vi "Log Folder.vi"(8 "error in (no error)":errorcluster, 11 "Node Config in":refnum<class "Node Config.lvclass">) -> (0 "error out":errorcluster, 2 "Log Folder":path, 3 "Node Config out":refnum<class "Node Config.lvclass">)   [LabVIEW 2020, in "VolatusConfig.lvlib" / "Node Config.lvclass"]
uses:
  Node Config.lvclass
  Node Config.lvclass/Node Config.ctl
  VolatusConfigElement/VolatusConfigElement.lvclass
  lv-cdm/CDM-Config/Config Element/Config Element.lvclass
  C:/dev/lv20CE/relink/lv-volatus/VolatusConfig/VolatusConfigElement/VolatusConfigElement.lvclass
  C:/dev/lv20CE/relink/lv-volatus/VolatusConfig/Node/Node Config.lvclass
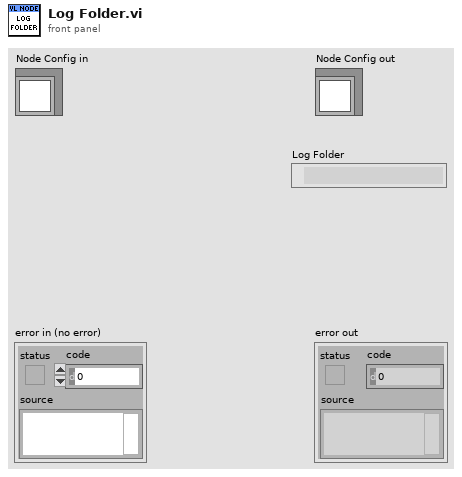
[diagram p1: front panel]
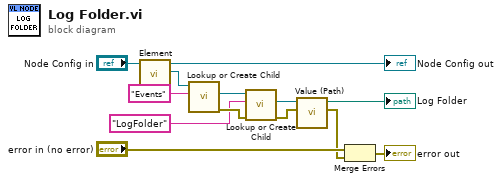
[diagram p0: block diagram]
diagram:
  n1 = call "Element.vi"("VolatusConfigElement in"="Node Config in") -> ("Element"=w12:refnum<class "Config Element.lvclass">, "VolatusConfigElement out"=→"Node Config out":refnum<class "Node Config.lvclass">)  [unwired: 9 in]
  n2 = call "Lookup or Create Child.vi"("Name"="Events", "Config Element in"=w12) -> ("error out"=w9:errorcluster, "Child"=w10:refnum<class "Config Element.lvclass">)  [unwired: 6 in, 2 out]
  n3 = call "Lookup or Create Child.vi"("error in (no error)"=w9, "Name"="LogFolder", "Config Element in"=w10) -> ("error out"=w7:errorcluster, "Child"=w6:refnum<class "Config Element.lvclass">)  [unwired: 5 in, 2 out]
  n4 = call "Value (Path).vi"("error in (no error)"=w7, "Config Element in"=w6) -> ("error out"=w1:errorcluster, "Path Value"=→"Log Folder":path)  [unwired: 8 in]
  n5 = Merge Errors("error in (no error)", w1) -> (→"error out":errorcluster)
